vi "test Message - Put Multiple.vi"(8 "error in (no error)":errorcluster, 11 "TestCase in":refnum<class "Test_Queue.lvclass">) -> (0 "error out":errorcluster, 3 "TestCase out":refnum<class "Test_Queue.lvclass">)   [LabVIEW 2015, in "Test_Queue.lvclass"]
uses:
  Test_Queue.lvclass
  Global Parameters.vi
  Core/Session/Session.lvclass
  Queue/NI_Azure_Queue.lvlib
  _shared/_Unit Tests Shared.lvlib
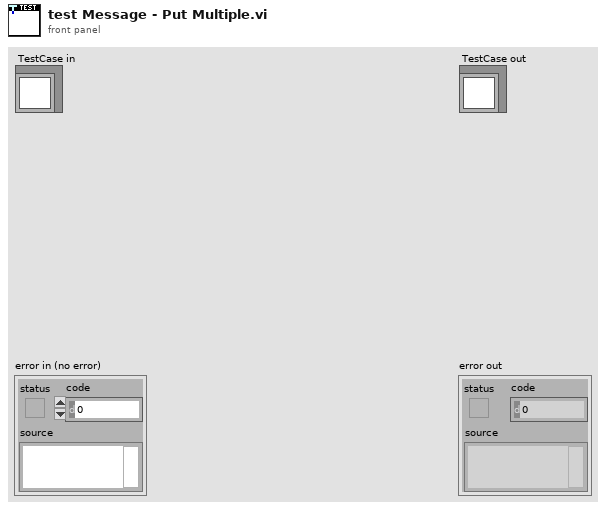
[diagram p1: front panel]
types:
  T1 = typedef "NI_Azure_Core.lvlib/Session.lvclass/Azure Credentials.ctl" = cluster{"Storage Account Name":string, "Access Key":string}
  T2 = typedef "NI_Azure_Queue.lvlib/Message.ctl" = cluster{"Message ID":string, "Insertion Time":string, "Expiration Time":string, "Pop Receipt":string, "Time Next Visible":string, "Dequeue Count":i32, "Message Text":string}
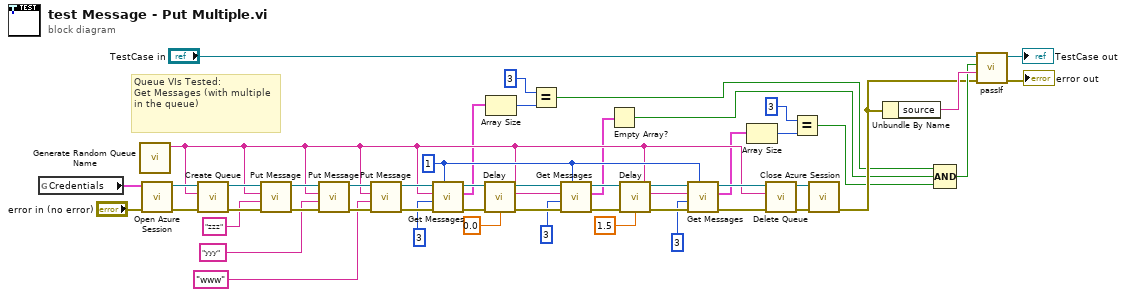
[diagram p0: block diagram]
diagram:
  w22 = u32 1 ("Visibility timeout (30 seconds)")
  # "Queue VIs Tested:\nGet Messages (with multiple in the queue)"
  n1 = global read "Global Parameters.vi" "Credentials"() -> (w42:T1)
  n2 = call "Generate Random Queue Name.vi"() -> ("Random Queue Name"=w14:string)  [unwired: 11 in]
  n3 = call "Open Azure Session.vi"("error in (no error)"="error in (no error)", "Credentials"=w42) -> ("error out"=w43:errorcluster, "Azure Session"=w38:refnum<class "Session.lvclass">)  [unwired: 8 in]
  n4 = call "Create Queue.vi"("error in (no error)"=w43, "Queue"=w14, "Azure Session in"=w38) -> ("error out"=w39:errorcluster, "Azure Session out"=w34:refnum<class "Session.lvclass">)  [unwired: 7 in]
  n5 = call "Put Message.vi"("error in (no error)"=w39, "Message"="zzz", "Queue"=w14, "Azure Session in"=w34) -> ("error out"=w35:errorcluster, "Azure Session out"=w20:refnum<class "Session.lvclass">)  [unwired: 5 in, 1 out]
  n6 = call "Put Message.vi"("error in (no error)"=w35, "Message"="yyy", "Queue"=w14, "Azure Session in"=w20) -> ("error out"=w21:errorcluster, "Azure Session out"=w17:refnum<class "Session.lvclass">)  [unwired: 5 in, 1 out]
  n7 = call "Put Message.vi"("error in (no error)"=w21, "Message"="www", "Queue"=w14, "Azure Session in"=w17) -> ("error out"=w18:errorcluster, "Azure Session out"=w16:refnum<class "Session.lvclass">)  [unwired: 5 in, 1 out]
  n8 = call "Get Messages.vi"("Visibility timeout (30 seconds)"=w22, "error in (no error)"=w18, "Number of messages (1)"=u32 3, "Queue"=w14, "Azure Session in"=w16) -> ("error out"=w29:errorcluster, "Messages"=w12:T2[], "Azure Session out"=w33:refnum<class "Session.lvclass">)  [unwired: 4 in]
  n9 = call "Delay.vi"("error in"=w29, "delay (1 sec)"=0.0) -> ("error out"=w28:errorcluster)  [unwired: 13 in]
  n10 = Array Size(array=w12) -> (size(s)=w11:i32)
  n11 = Equal?(x=3, y=w11) -> (x = y?=w3:bool)
  n12 = call "Get Messages.vi"("Visibility timeout (30 seconds)"=w22, "error in (no error)"=w28, "Number of messages (1)"=u32 3, "Queue"=w14, "Azure Session in"=w33) -> ("error out"=w25:errorcluster, "Messages"=w9:T2[], "Azure Session out"=w31:refnum<class "Session.lvclass">)  [unwired: 4 in]
  n13 = Empty Array?(array=w9) -> (empty?=w4:bool)
  n14 = call "Delay.vi"("error in"=w25, "delay (1 sec)"=1.5) -> ("error out"=w24:errorcluster)  [unwired: 13 in]
  n15 = call "Get Messages.vi"("Visibility timeout (30 seconds)"=w22, "error in (no error)"=w24, "Number of messages (1)"=u32 3, "Queue"=w14, "Azure Session in"=w31) -> ("error out"=w23:errorcluster, "Messages"=w6:T2[], "Azure Session out"=w30:refnum<class "Session.lvclass">)  [unwired: 4 in]
  n16 = Array Size(array=w6) -> (size(s)=w7:i32)
  n17 = call "Delete Queue.vi"("error in (no error)"=w23, "Queue"=w14, "Azure Session in"=w30) -> ("error out"=w37:errorcluster, "Azure Session out"=w36:refnum<class "Session.lvclass">)  [unwired: 7 in]
  n18 = Equal?(x=3, y=w7) -> (x = y?=w5:bool)
  n19 = call "Close Azure Session.vi"("error in (no error)"=w37, "Azure Session"=w36) -> ("error out"=w40:errorcluster)  [unwired: 9 in]
  n20 = Unbundle By Name(w40) -> ("source"=w45:string)
  n21 = Compound Arithmetic op=AND(w3, w4, w5) -> (w41:bool)
  n22 = call-dynamic "passIf.vi"("error in (no error)"=w40, "message (\"\")"=w45, "pass"=w41, "TestCase in"="TestCase in") -> ("error out"=→"error out":errorcluster, "TestCase out"=→"TestCase out":refnum<class "Test_Queue.lvclass">)  [unwired: 6 in]
